vi "System Battery Monitor.vi"(8 "Error In":errorcluster) -> (0 "Error Out":errorcluster)   [LabVIEW 2010]
uses:
  Windows/System32/kernel32.dll
panel:
  in  "Boolean":bool
  out "No System Battery":bool
  out "Estimated Time":string
  out "Charging":bool
  out "Critical":bool
  out "Low":bool
  out "High":bool
  out "DC Power":bool
  out "AC Power":bool
  out "Battery":u8(slide) scale=0.0..100.0
  in  "stop":bool
  # "System Power Monitor"
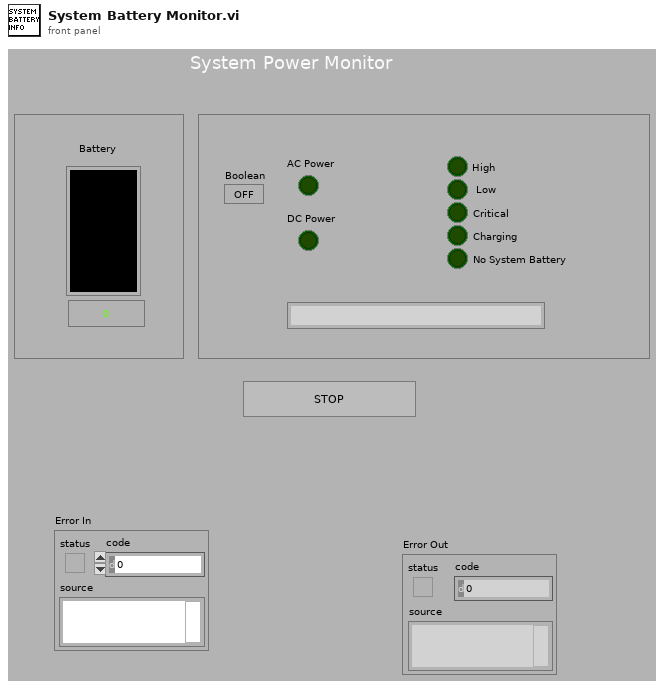
[diagram p1: front panel]
types:
  T1 = cluster{"ACLineStatus":u8, "BatteryFlag":u8, "BaterryLifePercent":u8, "Reserved":u8, "BatteryLifeTime":i32, "BatteryFullLifeTime":i32}
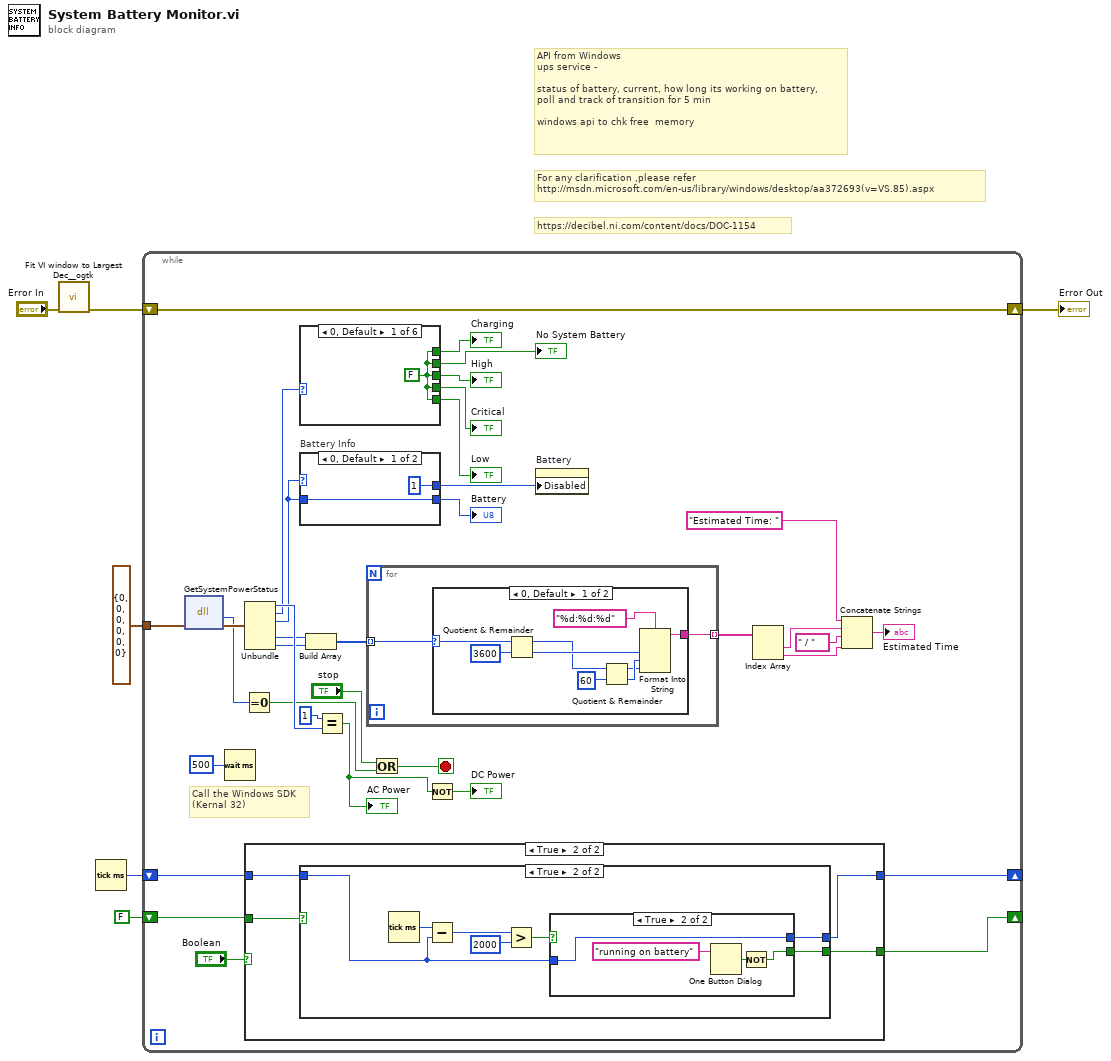
[diagram p0: block diagram]
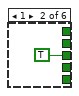
[diagram p5: hidden frame]
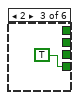
[diagram p6: hidden frame]
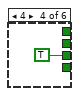
[diagram p7: hidden frame]
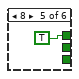
[diagram p8: hidden frame]
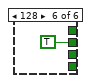
[diagram p9: hidden frame]
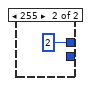
[diagram p10: hidden frame]
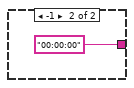
[diagram p11: hidden frame]
diagram:
  # "https://decibel.ni.com/content/docs/DOC-1154"
  # "API from Windows\nups service -\n\nstatus of battery, current, how long its working on battery, \npoll and track of transition for 5 min\n\nwindows api to chk free  memory"
  # "For any clarification ,please refer\nhttp://msdn.microsoft.com/en-us/library/windows/desktop/aa372693(v=VS.85).aspx"
  n1 = call <userlib>:"Fit VI window to Largest Dec__ogtk.vi"("error in (no error)"="Error In") -> ("error out"=w3:errorcluster)  [unwired: 5 in, 1 out]
  n2 = Tick Count (ms)() -> (millisecond timer value=w2:u32)
  n3 = while {
    shift-right: [w40] -> w6
    shift-left: w3 -> [w40]
    tunnel: T1 {"ACLineStatus"=0, "BatteryFlag"=0, "BaterryLifePercent"=0, "Reserved"=0, "BatteryLifeTime"=0, "BatteryFullLifeTime"=0} ("system_power_status") -> [w26]
    shift-right: [w11] -> _
    shift-left: w2 -> [w13]
    shift-right: [w12] -> _
    shift-left: FALSE ("DC Power") -> [w10]
    stop <- w25 stop-if-true
    # "Call the Windows SDK\n(Kernal 32)"
    n4 = dll-call lib="C:/Windows/System32/kernel32.dll" fn="GetSystemPowerStatus"("system_power_status"=w26) -> (w27:i32, "system_power_status"=w28:T1)  [unwired: 3 in, 2 out]
    n5 = Wait (ms)(milliseconds to wait=u32 500) -> ()  [unwired: 1 out]
    n6 = Equal To 0?(x=w27) -> (x = 0?=w24:bool)
    n7 = Unbundle(w28) -> ("ACLineStatus"=w39:u8, "BatteryFlag"=w22:u8, "BaterryLifePercent"=w16:u8, "BatteryLifeTime"=w31:i32, "BatteryFullLifeTime"=w32:i32)  [unwired: 1 out]
    n8 = case shown="True" "Boolean" {
      tunnel: w13 -> [_ w47]
      tunnel: w10 -> [_ w46]
      tunnel: [TRUE ("DC Power") w44] -> w12
      tunnel: [w42 w45] -> w11
      frame False {
        n9 = Tick Count (ms)() -> (millisecond timer value=w42:u32)
      }
      frame True {
        n10 = case shown="True" w46 {
          tunnel: w47 -> [w49 w51]
          tunnel: [w49 w53] -> w45
          tunnel: [FALSE ("DC Power") w50] -> w44
          frame False {
          }
          frame True {
            n11 = Tick Count (ms)() -> (millisecond timer value=w52:u32)
            n12 = Subtract(x=w52, y=w51) -> (x-y=w56:u32)
            n13 = Greater?(x=w56, y=u32 2000) -> (0:w54:bool)
            n14 = case shown="True" w54 {
              tunnel: [w58 w61] -> w53
              tunnel: w51 -> [w58 w61]
              tunnel: [TRUE w59] -> w50
              frame False {
              }
              frame True {
                n15 = One Button Dialog(message="running on battery") -> (true=w60:bool)  [unwired: 1 in]
                n16 = Not(x=w60) -> (.not. x?=w59:bool)
              }
            }
          }
        }
      }
    }
    n17 = case shown="0, Default" w22 {
      tunnel: [w63 TRUE ("High") _ _ _ _] -> w21
      tunnel: [w63 _ TRUE ("High") _ _ _] -> w20
      tunnel: [w63 _ _ TRUE ("High") _ _] -> w19
      tunnel: [w63 _ _ _ TRUE ("High") _] -> w18
      tunnel: [w63 _ _ _ _ TRUE ("High")] -> w17
      frame 0, Default {
        w63 = FALSE ("High")
      }
      frame 1 {
      }
      frame 2 {
      }
      frame 4 {
      }
      frame 8 {
      }
      frame 128 {
      }
    }
    "High" <- w21
    "Low" <- w20
    "Critical" <- w19
    "Charging" <- w18
    "No System Battery" <- w17
    n18 = case "Battery Info" shown="0, Default" w16 {
      tunnel: w16 -> [w70 _]
      tunnel: [w70 _] -> w15
      tunnel: [u8 1 ("Disabled") u8 2 ("Disabled")] -> w14
      frame 0, Default {
      }
      frame 255 {
      }
    }
    "Battery" <- w15
    n19 = Build Array(w31, w32) -> (w33:i32[])
    n20 = Equal?(x=u8 1 ("y"), y=w39) -> (x = y?=w9:bool)
    "AC Power" <- w9
    n21 = for {
      tunnel: w33 -> [w72] mode=indexing
      tunnel: [w73] -> w34 mode=indexing
      n22 = case shown="0, Default" w72 {
        selector: w72 -> [w78 _]
        tunnel: [w79 "00:00:00"] -> w73
        frame 0, Default {
          n23 = Quotient & Remainder(x=w78, y=3600) -> (x-y*floor(x/y)=w76:i32, floor(x/y)=w77:i32)
          n24 = Quotient & Remainder(x=w76, y=60) -> (x-y*floor(x/y)=w74:i32, floor(x/y)=w75:i32)
          n25 = Format Into String(format string="%d:%d:%d", w77, w75, w74) -> (resulting string=w79:string)  [unwired: 2 in, 1 out]
        }
        frame -1 {
        }
      }
    }
    n26 = Or(x="stop", y=w24) -> (x .or. y?=w25:bool)
    n27 = Not(x=w9) -> (.not. x?=→"DC Power":bool)
    n28 = property on="Battery" class="Slide (strict)"("Disabled"=w14) -> ()  [unwired: 2 in, 2 out]
    n29 = Index Array(array=w34) -> (element #1=w38:string, element #2=w35:string)  [unwired: 2 in]
    n30 = Concatenate Strings("Estimated Time: " ("format string"), w38, " / " ("format string"), w35) -> (→"Estimated Time":string)
  }
  "Error Out" <- w6
